vi "test_delete_and_readd_element.vi"() -> ()   [LabVIEW 2016]
uses:
  find_element(array).vi
  delete_element(variant).vi
panel:
  out "elapsed time in millisec (variant)":dbl
  out "elapsed time in millisec (array)":dbl
  in  "number of elements":i32=10000
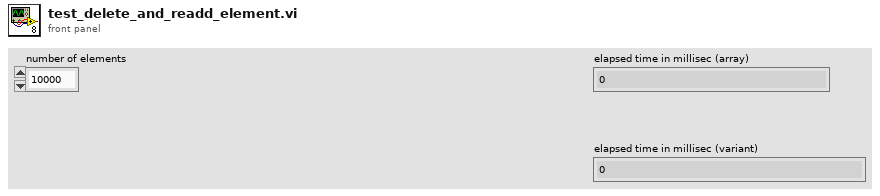
[diagram p1: front panel]
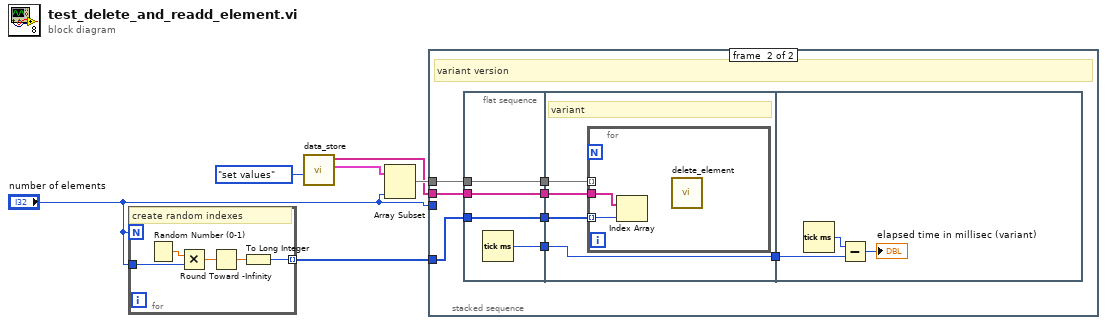
[diagram p0: block diagram]
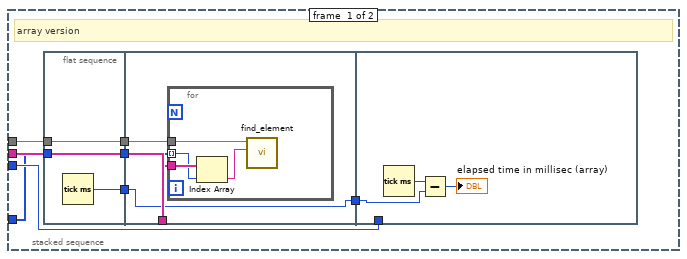
[diagram p2: hidden frame]
diagram:
  n1 = for {
    N: "number of elements" -> [_]
    tunnel: "number of elements" -> [w11]
    tunnel: [w7] -> w2 mode=indexing
    # "create random indexes"
    n2 = Random Number (0-1)() -> (number: 0 to 1=w10:dbl)
    n3 = Multiply(x=w10, y=w11) -> (x*y=w9:dbl)
    n4 = Round Toward -Infinity(1:w9) -> (0:w8:dbl)
    n5 = To Long Integer(number=w8) -> (32bit integer=w7:i32)
  }
  n6 = call "data_store.vi"("Action"=enum16{"set values", "get values"}."set values") -> ("array items"=w6:cluster{"name":string, "address":string}[], "names"=w3:string[])  [unwired: 9 in]
  n7 = Array Subset(array=w6, length="number of elements") -> (w5:cluster{"name":string, "address":string}[])  [unwired: 1 in]
  n8 = stacked-sequence {
    tunnel: "number of elements" -> [w16 _]
    tunnel: w5 -> [w15 w38]
    tunnel: w3 -> [w14 w35]
    tunnel: w2 -> [w13 w37]
    frame #0 {
      # "array version"
      n9 = flat-sequence {
        tunnel: [w22] -> w19
        tunnel: w15 -> [w21]
        tunnel: [w21] -> w18
        tunnel: w13 -> [w20]
        tunnel: [w20] -> w12
        tunnel: [w26] -> w17
        tunnel: w19 -> [w26]
        tunnel: w18 -> [w25]
        tunnel: w14 -> [w24]
        tunnel: w12 -> [w23]
        tunnel: w17 -> [w32]
        tunnel: w16 -> [_]
        frame #0 {
          n10 = Tick Count (ms)() -> (millisecond timer value=w22:u32)
        }
        frame #1 {
          n11 = for {
            tunnel: w25 -> [w28]
            tunnel: w24 -> [w30]
            tunnel: w23 -> [w29] mode=indexing
            n12 = Index Array(array=w30, index=w29) -> (element=w27:string)
            n13 = call-poly "find_element.vi"("name"=w27, "data store (in)"=w28) -> ()  [unwired: 6 in, 4 out]
          }
        }
        frame #2 {
          n14 = Tick Count (ms)() -> (millisecond timer value=w33:u32)
          n15 = Subtract(x=w33, y=w32) -> (x-y=→"elapsed time in millisec (array)":u32)
        }
      }
    }
    frame #1 {
      # "variant version"
      n16 = flat-sequence {
        tunnel: [w45] -> w41
        tunnel: w38 -> [w44]
        tunnel: [w44] -> w40
        tunnel: w37 -> [w43]
        tunnel: [w43] -> w36
        tunnel: w35 -> [w42]
        tunnel: [w42] -> w34
        tunnel: [w49] -> w39
        tunnel: w41 -> [w49]
        tunnel: w40 -> [w48]
        tunnel: w36 -> [w47]
        tunnel: w34 -> [w46]
        tunnel: w39 -> [w53]
        frame #0 {
          n17 = Tick Count (ms)() -> (millisecond timer value=w45:u32)
        }
        frame #1 {
          # "variant"
          n18 = for {
            tunnel: w48 -> [_] mode=indexing
            tunnel: w47 -> [w51] mode=indexing
            tunnel: w46 -> [w50]
            n19 = Index Array(array=w50, index=w51) -> ()  [unwired: 1 out]
            n20 = call-poly "delete_element.vi"() -> ()  [unwired: 9 in, 3 out]
          }
        }
        frame #2 {
          n21 = Tick Count (ms)() -> (millisecond timer value=w54:u32)
          n22 = Subtract(x=w54, y=w53) -> (x-y=→"elapsed time in millisec (variant)":u32)
        }
      }
    }
  }
